vi "MIO Get DC Level.vi"() -> (0 "DC Level":dbl format="%.3f")   [LabVIEW 2009]
uses:
  QCA Global.vi
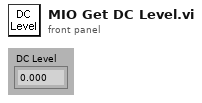
[diagram p1: front panel]
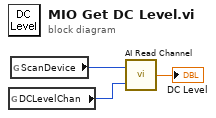
[diagram p0: block diagram]
diagram:
  n1 = global read "QCA Global.vi" "DCLevelChan"() -> (w2:i32)
  n2 = global read "QCA Global.vi" "ScanDevice"() -> (w3:i32)
  n3 = call "AI Read Channel.vi"("Channel"=w2, "Device"=w3) -> ("Value"=→"DC Level":dbl)
